vi "Main FPGA 5-axis with 5AxisLimitU8.vi"() -> ()   [LabVIEW 2013]
uses:
  <vilib>/Motion/MotorControl/_s/nism.interpretControlRegister.stateTransition.ctl
  <vilib>/Platform/TimedLoop/XDataNode/timing_clust.ctl
  <vilib>/Platform/TimedLoop/XDataNode/nitl_modes.ctl
  <vilib>/Platform/TimedLoop/XDataNode/wakeup.ctl
  <vilib>/Motion/MotorControl/_s/nism.digitalInputs.portA.ctl
  <vilib>/rvi/Emulation/niFpgaSctlEmulationGetInTimedLoop.vi
  <vilib>/rvi/Emulation/niFpgaEmulationReportErrorSimple.vi
  <vilib>/rvi/Emulation/niFpgaGetClockAttributes.vi
  <vilib>/rvi/Emulation/niFpgaCriticalErrorInLSC.vi
  Global FPGA.vi
  <vilib>/rvi/eio/common/nirviEmuTemplateMethod_errors.vi
  <vilib>/Motion/SoftMotion/Synchronization/nism.rioScan.generateSyncScan.vi
  <vilib>/rvi/Emulation/niFpgaProcessEmulError.vi
  <vilib>/Motion/MotorControl/_s/nism.interpretControlRegister.indexed.vi
  <vilib>/Motion/MotorControl/_s/nism.generateStatusRegister.indexed.vi
  <vilib>/Motion/MotorControl/_s/nism.mdo.read.positionLoopSyncData.vi
  <vilib>/Motion/MotorControl/_s/nism.mdo.read.splineData.vi
  <vilib>/Motion/MotorControl/_s/nism.splineInterpolation.fxp.3.index.vi
  <vilib>/Motion/MotorControl/_s/nism.mdo.handler.indexed.vi
  <vilib>/Motion/MotorControl/_s/nism.interpretDIOControl.portA.single.2.vi
  <vilib>/Motion/MotorControl/_s/nism.generateDIOStatus.portA.single.vi
  <vilib>/Platform/TimedLoop/XDataNode/XDataNode.xnode
  <vilib>/eio/EIONode/EIONode.xnode
  <vilib>/Motion/MotorControl/NI_SoftMotion_MotorControlIP.lvlib
  <vilib>/Platform/TimedLoop/XDataNode/XDNodeRunTimeDep.lvlib
  <vilib>/Motion/SoftMotion/Synchronization/NI_SoftMotion_Synchronization.lvlib
panel:
  in  "Axis Digital Input":u8[](array[numeric])=[0, 0, 0, 0, 0]
  out "Axis Positions":fxp<+/-,64,32>[](array[numeric])
  in  "STEP or CW? (T=STEP)":bool
  out "Drive Enable":bool[](array[boolean])
  in  "Enable Watchdog":bool
  in  "Pet Watchdog":bool
  in  "Watchdog Timeout Period (ticks)":u64=40000000 format="%.0p"
  out "Watchdog Timed Out?":bool
  out "Time Since Last Pet":u64
  in  "Enable value":bool
  in  "Drive Enable override?":bool
  out "State":T1=enum."Start --> Initializing" caption="state transition"
  in  "Sync Value":bool
  in  "Sync Enable override?":bool
  in  "Invert direction?":bool
  out "Sync is Fault":bool
  out "Sync is Locked":bool
  in  "minimum pulse":u16=40
  # "Synchronization Loop"
  # "Control Status Loop"
  # "Notes: \n1. This VI provides the communication interface between the NI SoftMotion Engine and the LabVIEW FPGA Module. You must compile this VI for a specific FPGA target before use. After compiling, run the VI before running any of the Express VI examples. For information on moving this example to another FPGA target, refer to ni.com/info and enter info code fpgaex.\n\n2. Only use the Reset Axis button if you are unable to communicate with the axis by any other means. This button resets the device state machine and other VIs to a known state. After resetting the axis, switch the NI Scan Engine from Active Mode to Configuration Mode, then back to Active Mode, before attempting to enable the axis."
  # "(These two buttons \nare for testing\npurposes.)"
  # "(These two buttons \nare for testing\npurposes.)"
  # "Step/Direction Loop"
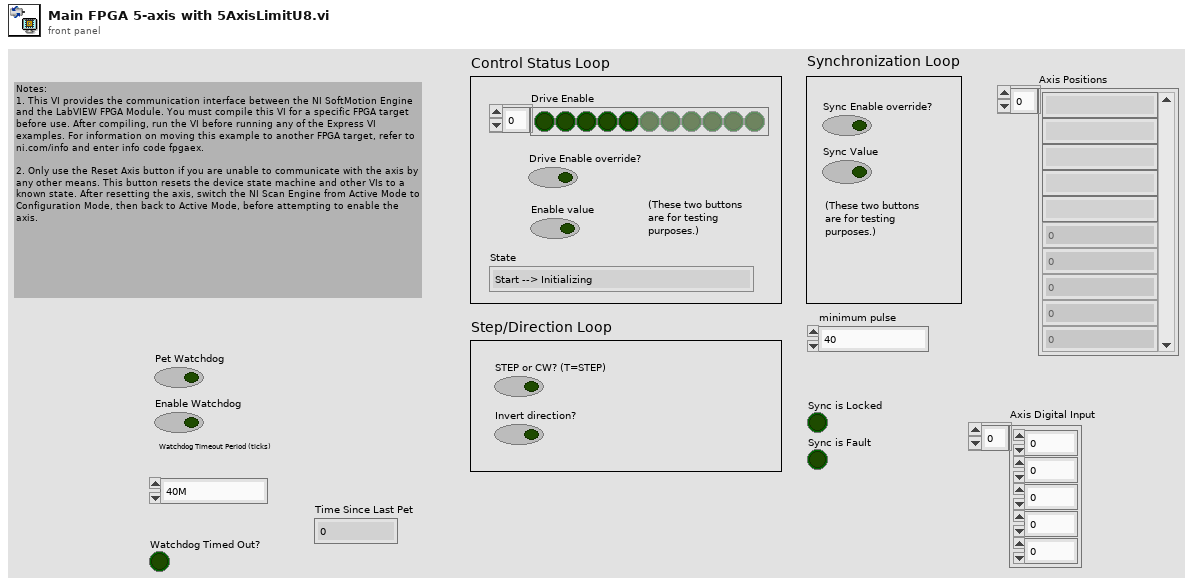
[diagram p1: front panel]
types:
  T1 = typedef "NI_SoftMotion_MotorControlIP.lvlib/nism.interpretControlRegister.stateTransition.ctl" = enum8{"Invalid", "Start --> Initializing", "Initializing --> Disabled", "Disabled --> Ready To Switch On", "Ready To Switch On --> Switched On", "Ready To Switch On --> Disable", "Switched On --> Operation Enable", "Switched On --> Ready To Switch On", "Switched On --> Disabled", "Operation Enable --> Switched On", "Operation Enable --> Ready To Switch On", "Operation Enable --> Disabled", "Fault --> Disabled", "Any --> Fault", "None"}
  T2 = typedef "NI_SoftMotion_MotorControlIP.lvlib/nism.mdo.splineData.ctl" = cluster{"spline type":T3, "traj per/spline per":u16, "spline per/traj per":fxp<+,32,0>}
  T3 = typedef "nism.splineInterpolation.type.ctl" = u16
  T4 = typedef "NI_SoftMotion_Synchronization.lvlib/nism.softmotionScan.timerConfig.ctl" = cluster{"Target Period (clocks)":u16, "Host Period / Target Period":u16}
  T5 = typedef "NI_SoftMotion_MotorControlIP.lvlib/nism.digitalInputs.portA.ctl" = cluster{"reverse limit":bool, "forward limit":bool, "home switch":bool, "digital input 0":bool, "digital input 1":bool, "digital input 2":bool, "digital input 3":bool}
  T6 = typedef "NI_SoftMotion_MotorControlIP.lvlib/nism.dio.portA.config.2.ctl" = cluster{"digital filter (us)":u16[], "safe state":enum16{"Low", "High", "No Change"}[]}
  T7 = typedef "NI_SoftMotion_Synchronization.lvlib/nism.softmotionScan.timerControl.ctl" = cluster{"SM Scan":bool, "SM Scan Count":u32, "SM Scan Enabled":bool}
  T8 = typedef "XDNodeRunTimeDep.lvlib/timing_clust.ctl" = cluster{"Expected End [f-1]":u64, "Actual End [f-1]":u64, "Finished Late? [f-1]":bool, "Expected End [i-1]":u64, "Actual End [i-1]":u64, "Finished Late? [i-1]":bool, "Expected Start [i]":u64, "Actual Start [i]":u64, "Expected Start [f]":u64, "Actual Start [f]":u64, "Source Name":string, "Structure Name":string, "Period":i64, "Deadline":i64, "Offset":i64, "Start":i64, "Priority":i32, "Timeout":i32, "Mode":T9, "Wakeup Reason":T10, "Error":errorcluster, "Source Type":string, "Secondary Source Type":string, "Global End Time":u64, "Global Start Time":u64, "Frame Duration":u64, "Iteration Duration":u64, "Assigned CPU":i32, "I/O Scan Engine Mode":u32}
  T9 = typedef "XDNodeRunTimeDep.lvlib/nitl_modes.ctl" = enum32{"No Change", "Process missed periods, maintain original phase", "Discard missed periods, maintain original phase", "Process missed periods, ignore original phase", "Discard missed periods, ignore original phase"}
  T10 = typedef "XDNodeRunTimeDep.lvlib/wakeup.ctl" = enum32{"Normal", "Aborted", "Asynchronous wakeup", "Timing source error", "Timed loop error", "Timeout"}
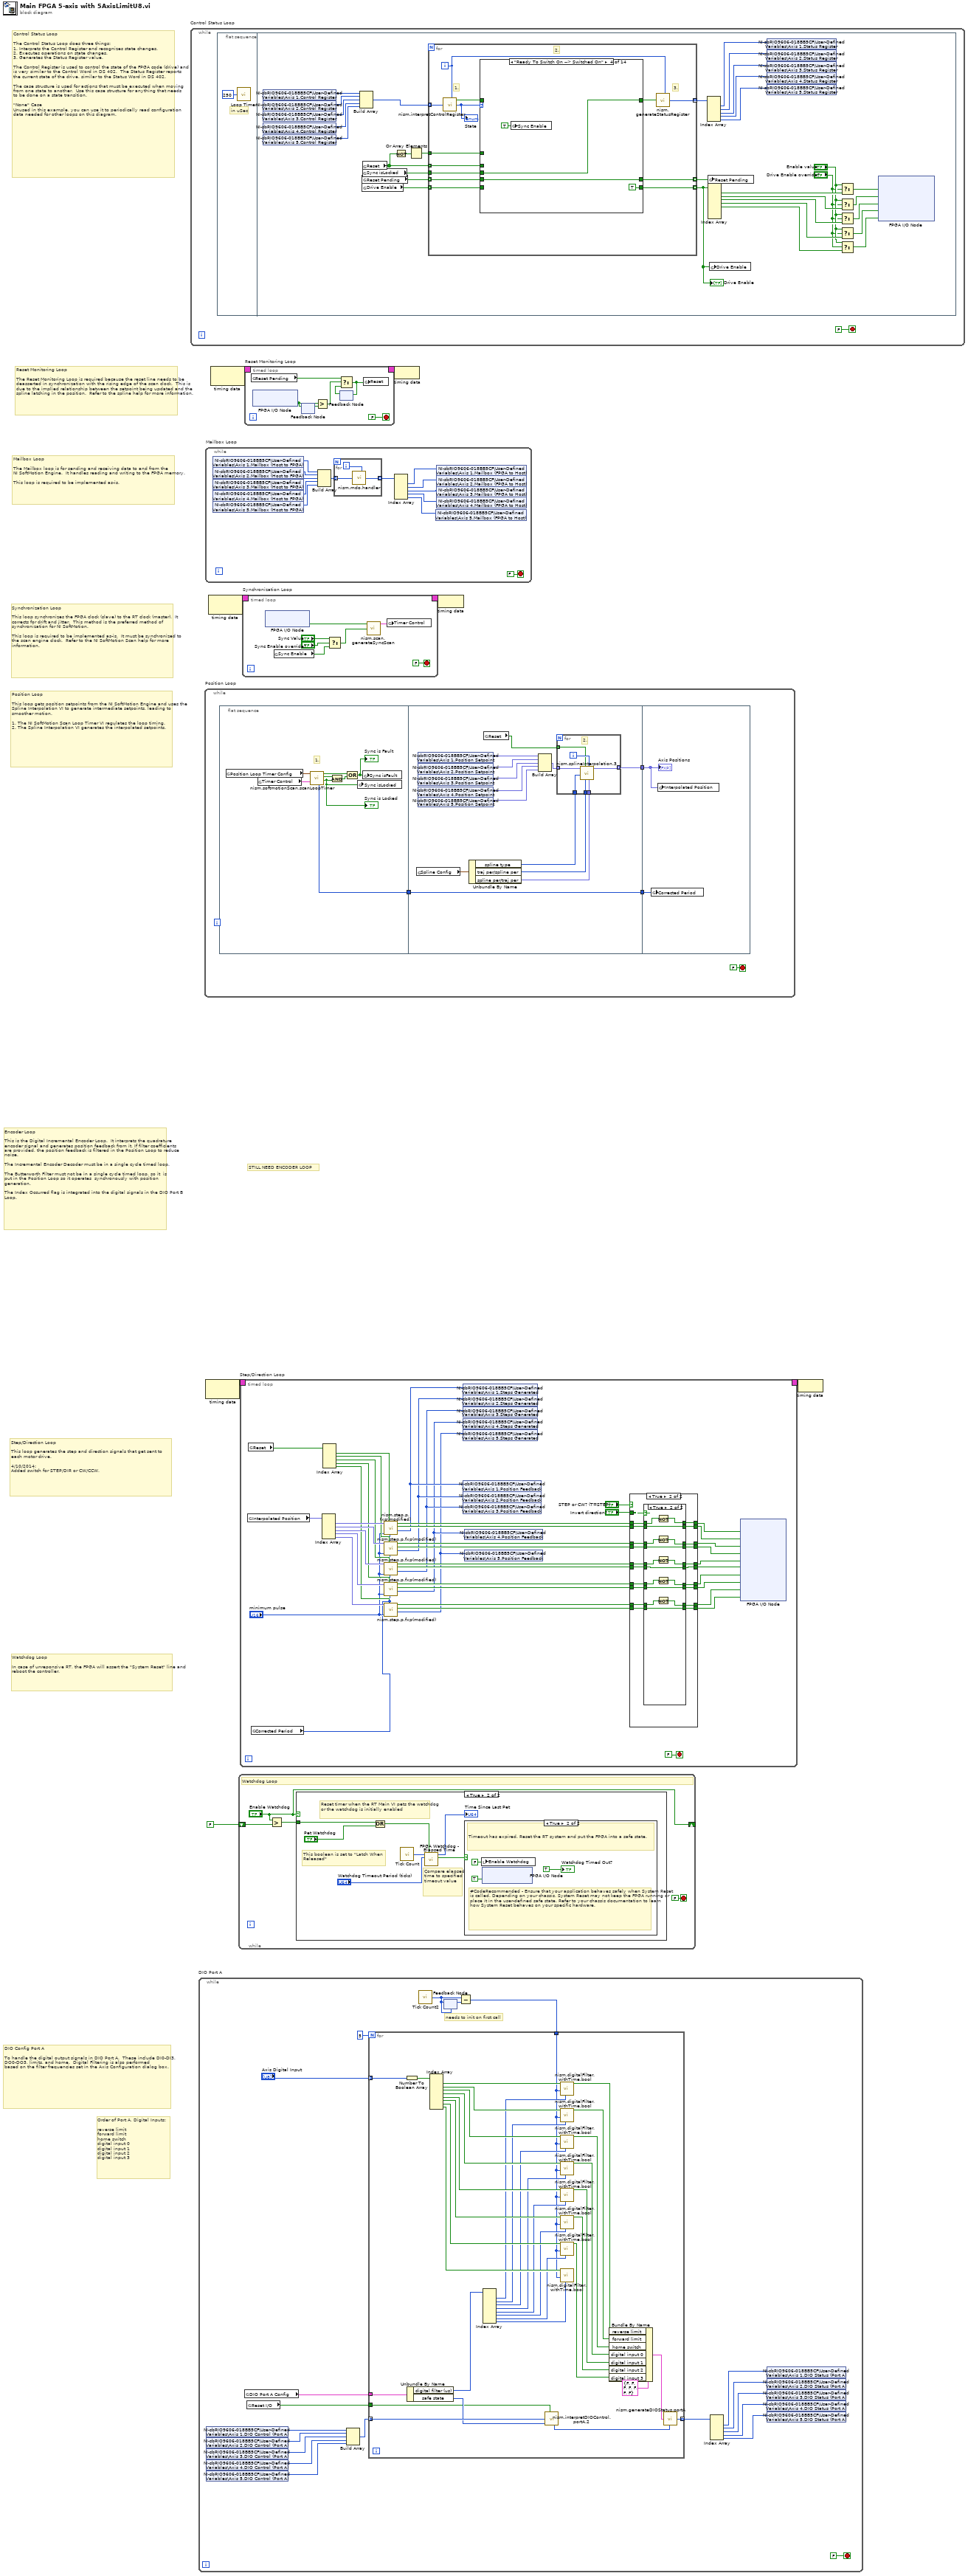
[diagram p0: block diagram]
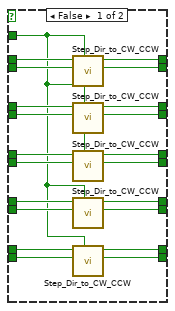
[diagram p4: hidden frame]
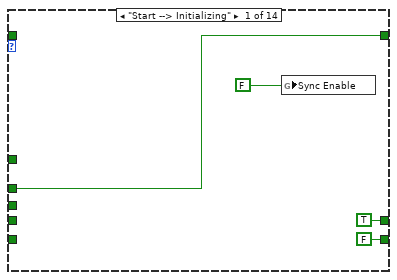
[diagram p6: hidden frame]
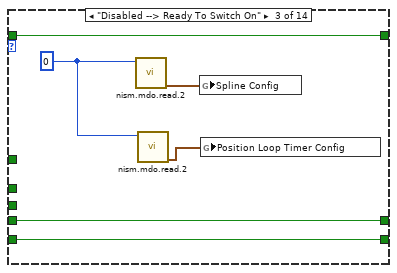
[diagram p8: hidden frame]
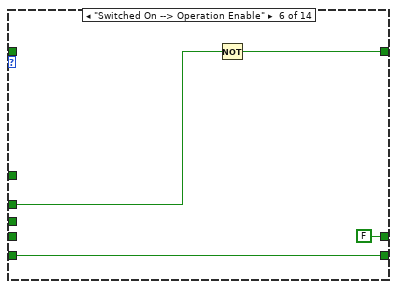
[diagram p10: hidden frame]
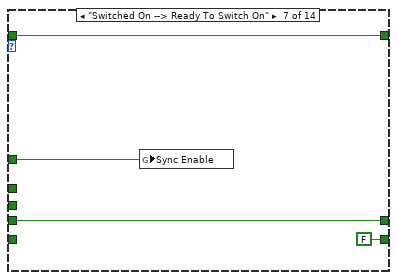
[diagram p11: hidden frame]
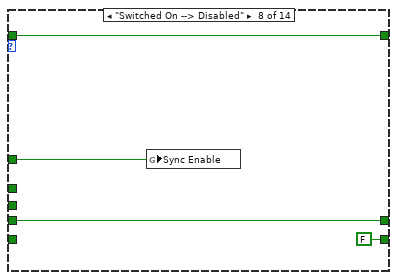
[diagram p12: hidden frame]
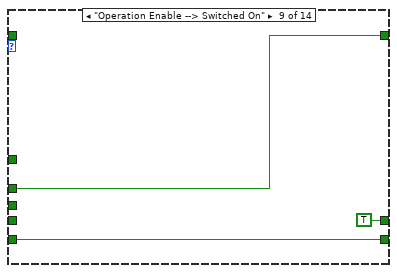
[diagram p13: hidden frame]
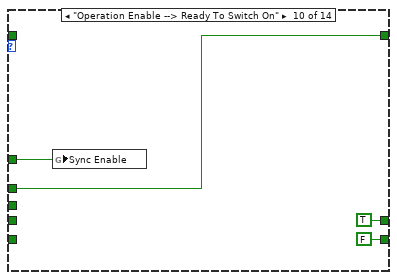
[diagram p14: hidden frame]
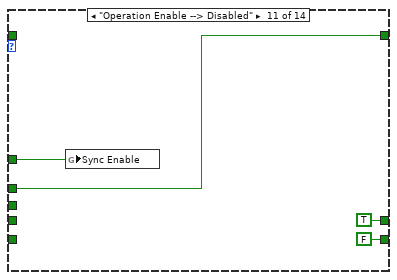
[diagram p15: hidden frame]
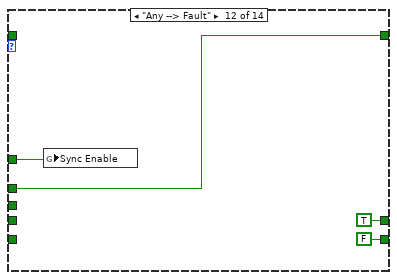
[diagram p16: hidden frame]
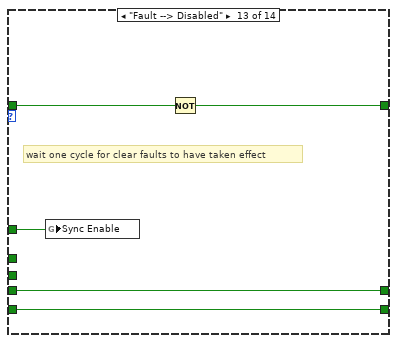
[diagram p17: hidden frame]
diagram:
  # "STILL NEED ENCODER LOOP"
  # "DIO Config Port A\n\nTo handle the digital output signals in DIO Port A.  These include DI0-DI3, DO0-DO3, limits, and home.  Digital Filtering is also performed\nbased on the filter frequencies set in the Axis Configuration dialog box."
  # "Order of Port A, Digital Inputs:\n\nreverse limit\nforward limit\nhome switch\ndigital input 0\ndigital input 1\ndigital input 2\ndigital input 3"
  # "Encoder Loop\n\nThis is the Digital Incremental Encoder Loop.  It interprets the quadrature encoder signal and generates position feedback from it. If filter coefficients are provided, the position feedback is filtered in the Position Loop to reduce noise.\n\nThe Incremental Encoder Decoder must be in a single cycle timed loop.\n\nThe Butterworth Filter must not be in a single cycle timed loop, so it  is\nput in the Position Loop so it operates  synchronously with position generation.\n\nThe Index Occurred flag is integrated into the digital signals in the DIO Port B Loop."
  # "Watchdog Loop\n\nIn case of unreponsive RT, the FPGA will assert the \"System Reset\" line and reboot the controller."
  # "Step/Direction Loop\n\nThis loop generates the step and direction signals that get sent to \neach motor drive.\n\n4/10/2014:\nAdded switch for STEP/DIR or CW/CCW."
  # "Position Loop\n\nThis loop gets position setpoints from the NI SoftMotion Engine and uses the Spline Interpolation VI to generate intermediate setpoints, leading to smoother motion.\n\n1. The NI SoftMotion Scan Loop Timer VI regulates the loop timing. \n2. The Spline Interpolation VI generates the interpolated setpoints."
  # "Synchronization Loop\n\nThis loop synchronizes the FPGA clock (slave) to the RT clock (master).  It corrects for drift and jitter.  This method is the preferred method of synchronization for NI SoftMotion.\n\nThis loop is required to be implemented as-is.  It must be synchronized to the scan engine clock.  Refer to the NI SoftMotion Scan help for more information."
  # "Mailbox Loop\n\nThe Mailbox loop is for sending and receiving data to and from the \nNI SoftMotion Engine.  It handles reading and writing to the FPGA memory.\n\nThis loop is required to be implemented as-is."
  # "Reset Monitoring Loop\n\nThe Reset Monitoring Loop is required because the reset line needs to be deasserted in synchronization with the rising edge of the scan clock.  This is due to the implied relationship between the setpoint being updated and the spline latching in the position.  Refer to the spline help for more information."
  # "Control Status Loop\n\nThe Control Status Loop does three things:\n1. Interprets the Control Register and recognizes state changes.\n2. Executes operations on state changes.\n3. Generates the Status Register value.\n\nThe Control Register is used to control the state of the FPGA code (drive) and is very similar to the Control Word in DS 402.  The Status Register reports the current state of the drive, similar to the Status Word in DS 402.\n\nThe case structure is used for actions that must be executed when moving from one state to another.  Use this case structure for anything that needs to be done on a state transition.\n\n\"None\" Case\nUnused in this example, you can use it to periodically read configuration data needed for other loops on this diagram."
  n1 = while "Control Status Loop" {
    stop <- FALSE stop-if-true
    n2 = flat-sequence {
      frame #0 {
        # "in uSec"
        n3 = call "Loop Timer"("Count(uSec)"=u32 250) -> ()  [unwired: 1 out]
      }
      frame #1 {
        n4 = shared-variable "NI-sbRIO9606-018BB5CF\\User-Defined Variables\\Axis 1.Control Register"() -> (w31:u32)  [unwired: 1 in, 1 out]
        n5 = shared-variable "NI-sbRIO9606-018BB5CF\\User-Defined Variables\\Axis 2.Control Register"() -> (w30:u32)  [unwired: 1 in, 1 out]
        n6 = shared-variable "NI-sbRIO9606-018BB5CF\\User-Defined Variables\\Axis 3.Control Register"() -> (w29:u32)  [unwired: 1 in, 1 out]
        n7 = shared-variable "NI-sbRIO9606-018BB5CF\\User-Defined Variables\\Axis 4.Control Register"() -> (w28:u32)  [unwired: 1 in, 1 out]
        n8 = shared-variable "NI-sbRIO9606-018BB5CF\\User-Defined Variables\\Axis 5.Control Register"() -> (w27:u32)  [unwired: 1 in, 1 out]
        n9 = Build Array(w31, w30, w29, w28, w27) -> (w40:u32[])
        n10 = global read "Global FPGA.vi" "Reset Pending"() -> (w35:bool[])
        n11 = global read "Global FPGA.vi" "Drive Enable"() -> (w34:bool[])
        n12 = global read "Global FPGA.vi" "Reset"() -> (w36:bool[])
        n13 = global read "Global FPGA.vi" "Sync isLocked"() -> (w41:bool)
        n14 = Not(x=w36) -> (.not. x?=w38:bool[])
        n15 = Or Array Elements(Boolean array=w38) -> (logical OR=w37:bool)
        n16 = for {
          tunnel: w36 -> [w49] mode=indexing
          tunnel: w41 -> [w48]
          tunnel: w40 -> [w50] mode=indexing
          tunnel: [w47] -> w32 mode=indexing
          tunnel: [w46] -> w39 mode=indexing
          tunnel: [w45] -> w33 mode=indexing
          tunnel: w37 -> [w44]
          tunnel: w35 -> [w43] mode=indexing
          tunnel: w34 -> [w42] mode=indexing
          i -> [w51]
          # "3."
          # "2."
          # "1."
          n17 = call-poly <vilib>:"nism.interpretControlRegister.vi"("control register"=w50, "axis index"=w51) -> ("transition occurred"=w52:bool, "state transition"=w53:T1)  [unwired: 6 in]
          "State" <- w53
          n18 = case shown="\"Ready To Switch On --> Switched On\"" w53 {
            tunnel: w52 -> [_ w61 w67 _ w74 _ w82 w86 _ _ _ _ w106 _]
            tunnel: [w58 w61 w67 w69 w74 w78 w82 w86 w88 w91 w95 w99 w105 _] -> w54
            tunnel: w49 -> [w58 _ _ _ _ w77 _ _ w88 w91 w95 w99 _ _]
            tunnel: w48 -> [_ _ _ w69 _ _ _ _ _ _ _ _ _ _]
            tunnel: [TRUE ("Write.Reset Pending") w60 w63 w68 w73 FALSE ("Write.Reset Pending") w79 w83 TRUE ("Write.Reset Pending") TRUE ("Write.Reset Pending") TRUE ("Write.Reset Pending") TRUE ("Write.Reset Pending") w103 w108] -> w46
            tunnel: [FALSE ("Write.Drive Enable") w59 w62 TRUE ("Write.Drive Enable") w72 w75 FALSE ("Write.Drive Enable") FALSE ("Write.Drive Enable") w87 FALSE ("Write.Drive Enable") FALSE ("Write.Drive Enable") FALSE ("Write.Drive Enable") w102 w107] -> w45
            tunnel: w44 -> [_ _ _ _ _ _ w80 w84 _ w90 w94 w98 w104 _]
            tunnel: w43 -> [_ w60 w63 w68 w73 _ w79 w83 _ _ _ _ w103 w108]
            tunnel: w42 -> [_ w59 w62 _ w72 w75 _ _ w87 _ _ _ w102 w107]
            frame "Start --> Initializing" {
              n19 = global write "Global FPGA.vi" "Sync Enable"(FALSE ("Sync Enable")) -> ()
            }
            frame "Initializing --> Disabled" {
            }
            frame "Disabled --> Ready To Switch On" {
              w65 = 0 ("axis index")
              n20 = call-poly <vilib>:"nism.mdo.read.2.vi"("axis index"=w65) -> ("spline"=w66:T2)  [unwired: 10 in]
              n21 = call-poly <vilib>:"nism.mdo.read.2.vi"("axis index"=w65) -> ("position loop sync"=w64:T4)  [unwired: 10 in]
              n22 = global write "Global FPGA.vi" "Spline Config"(w66) -> ()
              n23 = global write "Global FPGA.vi" "Position Loop Timer Config"(w64) -> ()
            }
            frame "Ready To Switch On --> Switched On" {
              n24 = global write "Global FPGA.vi" "Sync Enable"(TRUE ("Sync Enable")) -> ()
            }
            frame "Ready To Switch On --> Disable" {
            }
            frame "Switched On --> Operation Enable" {
              n25 = Not(x=w77) -> (.not. x?=w78:bool)
            }
            frame "Switched On --> Ready To Switch On" {
              n26 = global write "Global FPGA.vi" "Sync Enable"(w80) -> ()
            }
            frame "Switched On --> Disabled" {
              n27 = global write "Global FPGA.vi" "Sync Enable"(w84) -> ()
            }
            frame "Operation Enable --> Switched On" {
            }
            frame "Operation Enable --> Ready To Switch On" {
              n28 = global write "Global FPGA.vi" "Sync Enable"(w90) -> ()
            }
            frame "Operation Enable --> Disabled" {
              n29 = global write "Global FPGA.vi" "Sync Enable"(w94) -> ()
            }
            frame "Any --> Fault" {
              n30 = global write "Global FPGA.vi" "Sync Enable"(w98) -> ()
            }
            frame "Fault --> Disabled" {
              # "wait one cycle for clear faults to have taken effect"
              n31 = global write "Global FPGA.vi" "Sync Enable"(w104) -> ()
              n32 = Not(x=w106) -> (.not. x?=w105:bool)
            }
            frame "None", Default {
            }
          }
          n33 = call-poly <vilib>:"nism.generateStatusRegister.vi"("transition success"=w54, "axis index"=w51) -> ("status register"=w47:u32)  [unwired: 7 in]
        }
        "Drive Enable" <- w33
        n34 = Index Array(array=w32) -> (element #1=w26:u32, element #2=w25:u32, element #3=w24:u32, element #4=w23:u32, element #5=w22:u32)  [unwired: 5 in]
        n35 = global write "Global FPGA.vi" "Reset Pending"(w39) -> ()
        n36 = Index Array(array=w33) -> (element #1=w21:bool, element #2=w19:bool, element #3=w17:bool, element #4=w15:bool, element #5=w13:bool)  [unwired: 8 in, 3 out]
        n37 = global write "Global FPGA.vi" "Drive Enable"(w33) -> ()
        n38 = shared-variable "NI-sbRIO9606-018BB5CF\\User-Defined Variables\\Axis 1.Status Register"(w26) -> ()  [unwired: 1 in, 1 out]
        n39 = shared-variable "NI-sbRIO9606-018BB5CF\\User-Defined Variables\\Axis 2.Status Register"(w25) -> ()  [unwired: 1 in, 1 out]
        n40 = shared-variable "NI-sbRIO9606-018BB5CF\\User-Defined Variables\\Axis 3.Status Register"(w24) -> ()  [unwired: 1 in, 1 out]
        n41 = shared-variable "NI-sbRIO9606-018BB5CF\\User-Defined Variables\\Axis 4.Status Register"(w23) -> ()  [unwired: 1 in, 1 out]
        n42 = shared-variable "NI-sbRIO9606-018BB5CF\\User-Defined Variables\\Axis 5.Status Register"(w22) -> ()  [unwired: 1 in, 1 out]
        n43 = Select(t="Enable value", s="Drive Enable override?", f=w21) -> (s? t:f=w20:bool)
        n44 = Select(t="Enable value", s="Drive Enable override?", f=w19) -> (s? t:f=w18:bool)
        n45 = Select(t="Enable value", s="Drive Enable override?", f=w17) -> (s? t:f=w16:bool)
        n46 = Select(t="Enable value", s="Drive Enable override?", f=w15) -> (s? t:f=w14:bool)
        n47 = Select(t="Enable value", s="Drive Enable override?", f=w13) -> (s? t:f=w12:bool)
        n48 = xnode "FPGA I/O Node"("Axis1_Servo On"=w20, "Axis2_Servo On"=w18, "Axis3_Servo On"=w16, "Axis4_Servo On"=w14, "Axis5_Servo On"=w12) -> ()  [unwired: 5 in, 5 out]
      }
    }
  }
  n49 = while "DIO Port A" {
    stop <- FALSE stop-if-true
    # "needs to init on first call"
    n50 = shared-variable "NI-sbRIO9606-018BB5CF\\User-Defined Variables\\Axis 1.DIO Control (Port A)"() -> (w123:u32)  [unwired: 1 in, 1 out]
    n51 = shared-variable "NI-sbRIO9606-018BB5CF\\User-Defined Variables\\Axis 2.DIO Control (Port A)"() -> (w122:u32)  [unwired: 1 in, 1 out]
    n52 = shared-variable "NI-sbRIO9606-018BB5CF\\User-Defined Variables\\Axis 3.DIO Control (Port A)"() -> (w121:u32)  [unwired: 1 in, 1 out]
    n53 = shared-variable "NI-sbRIO9606-018BB5CF\\User-Defined Variables\\Axis 4.DIO Control (Port A)"() -> (w120:u32)  [unwired: 1 in, 1 out]
    n54 = shared-variable "NI-sbRIO9606-018BB5CF\\User-Defined Variables\\Axis 5.DIO Control (Port A)"() -> (w119:u32)  [unwired: 1 in, 1 out]
    n55 = global read "Global FPGA.vi" "DIO Port A Config"() -> (w127:T6)
    n56 = global read "Global FPGA.vi" "Reset I/O"() -> (w126:bool)
    n57 = Build Array(w123, w122, w121, w120, w119) -> (w118:u32[])
    n58 = call "Tick Count2"() -> ("Tick Count(uSec)"=w111:u16)
    n59 = feedback #1(w111) -> (w110:u16)
    n60 = feedback-in #1(w111) -> ()
    n61 = Subtract(x=w111, y=w110) -> (x-y=w109:u16)
    n62 = for {
      N: 5 -> [_]
      tunnel: [w162] -> w112 mode=indexing
      tunnel: w118 -> [w161] mode=indexing
      tunnel: w127 -> [w158]
      tunnel: w126 -> [w156]
      tunnel: "Axis Digital Input" -> [w130] mode=indexing
      tunnel: w109 -> [w129]
      n63 = Number To Boolean Array(number=w130) -> (Boolean array=w155:bool[])
      n64 = Unbundle By Name(w158) -> ("digital filter (us)"=w138:u16[], "safe state"=w157:enum16{"Low", "High", "No Change"}[])
      n65 = Index Array(array=w155) -> (element #1=w154:bool, element #2=w147:bool, element #3=w148:bool, element #4=w149:bool, element #5=w150:bool, element #6=w151:bool, element #7=w152:bool, element #8=w153:bool)  [unwired: 8 in]
      n66 = Index Array(array=w138) -> (element #1=w139:u16, element #2=w140:u16, element #3=w141:u16, element #4=w142:u16, element #5=w143:u16, element #6=w144:u16, element #7=w145:u16, element #8=w146:u16)  [unwired: 8 in]
      n67 = call-poly <vilib>:"nism.interpretDIOControl.portA.2.vi"("reset"=w156, "dio control(port a)"=w161, "safe state"=w157) -> ("reset latches"=w163:u8)  [unwired: 5 in, 1 out]
      n68 = call <vilib>:"nism.digitalFilter.withTime.bool.vi"("filter value"=w139, "delta time"=w129, "input signal"=w154) -> ("output signal"=w137:bool)  [unwired: 8 in]
      n69 = call <vilib>:"nism.digitalFilter.withTime.bool.vi"("filter value"=w140, "delta time"=w129, "input signal"=w147) -> ("output signal"=w136:bool)  [unwired: 8 in]
      n70 = call <vilib>:"nism.digitalFilter.withTime.bool.vi"("filter value"=w141, "delta time"=w129, "input signal"=w148) -> ("output signal"=w135:bool)  [unwired: 8 in]
      n71 = call <vilib>:"nism.digitalFilter.withTime.bool.vi"("filter value"=w142, "delta time"=w129, "input signal"=w149) -> ("output signal"=w134:bool)  [unwired: 8 in]
      n72 = call <vilib>:"nism.digitalFilter.withTime.bool.vi"("filter value"=w143, "delta time"=w129, "input signal"=w150) -> ("output signal"=w133:bool)  [unwired: 8 in]
      n73 = call <vilib>:"nism.digitalFilter.withTime.bool.vi"("filter value"=w144, "delta time"=w129, "input signal"=w151) -> ("output signal"=w132:bool)  [unwired: 8 in]
      n74 = call <vilib>:"nism.digitalFilter.withTime.bool.vi"("filter value"=w145, "delta time"=w129, "input signal"=w152) -> ("output signal"=w131:bool)  [unwired: 8 in]
      n75 = call <vilib>:"nism.digitalFilter.withTime.bool.vi"("filter value"=w146, "delta time"=w129, "input signal"=w153) -> ()  [unwired: 8 in, 1 out]
      n76 = Bundle By Name(cluster=T5 {"reverse limit"=FALSE, "forward limit"=FALSE, "home switch"=FALSE, "digital input 0"=FALSE, "digital input 1"=FALSE, "digital input 2"=FALSE, "digital input 3"=FALSE} ("$(driveInterface.digitalInputs.shortName)"), "reverse limit"=w137, "forward limit"=w136, "home switch"=w135, "digital input 0"=w134, "digital input 1"=w133, "digital input 2"=w132, "digital input 3"=w131) -> (w159:T5)
      n77 = call-poly <vilib>:"nism.generateDIOStatus.portA.vi"("digital inputs"=w159, "reset latches"=w163) -> ("dio status(port a)"=w162:u32)  [unwired: 7 in]
    }
    n78 = Index Array(array=w112) -> (element #1=w117:u32, element #2=w116:u32, element #3=w115:u32, element #4=w114:u32, element #5=w113:u32)  [unwired: 5 in]
    n79 = shared-variable "NI-sbRIO9606-018BB5CF\\User-Defined Variables\\Axis 1.DIO Status (Port A)"(w117) -> ()  [unwired: 1 in, 1 out]
    n80 = shared-variable "NI-sbRIO9606-018BB5CF\\User-Defined Variables\\Axis 2.DIO Status (Port A)"(w116) -> ()  [unwired: 1 in, 1 out]
    n81 = shared-variable "NI-sbRIO9606-018BB5CF\\User-Defined Variables\\Axis 3.DIO Status (Port A)"(w115) -> ()  [unwired: 1 in, 1 out]
    n82 = shared-variable "NI-sbRIO9606-018BB5CF\\User-Defined Variables\\Axis 4.DIO Status (Port A)"(w114) -> ()  [unwired: 1 in, 1 out]
    n83 = shared-variable "NI-sbRIO9606-018BB5CF\\User-Defined Variables\\Axis 5.DIO Status (Port A)"(w113) -> ()  [unwired: 1 in, 1 out]
  }
  n84 = while "Position Loop" {
    stop <- FALSE stop-if-true
    n85 = flat-sequence {
      tunnel: [w168] -> w164
      tunnel: [w182] -> w166
      tunnel: [w181] -> w165
      tunnel: w164 -> [w181]
      tunnel: w166 -> [w196]
      tunnel: w165 -> [w197]
      frame #0 {
        # "1."
        n86 = global read "Global FPGA.vi" "Position Loop Timer Config"() -> (w170:T4)
        n87 = global read "Global FPGA.vi" "Timer Control"() -> (w169:T7)
        n88 = call <vilib>:"nism.softmotionScan.scanLoopTimer.vi"("Timer Control"=w169, "Timer Config"=w170) -> ("Scan Running?"=w172:bool, "Finished Late?"=w174:bool, "Fault Occurred?"=w175:bool, "Corrected Period"=w168:u16)  [unwired: 5 in, 1 out]
        "Sync is Locked" <- w172
        n89 = Compound Arithmetic op=AND(w174, w172) -> (w173:bool)
        n90 = Compound Arithmetic op=OR(w175, w173) -> (w171:bool)
        "Sync is Fault" <- w171
        n91 = global write "Global FPGA.vi" "Sync isLocked"(w172) -> ()
        n92 = global write "Global FPGA.vi" "Sync isFault"(w171) -> ()
      }
      frame #1 {
        n93 = global read "Global FPGA.vi" "Spline Config"() -> (w184:T2)
        n94 = shared-variable "NI-sbRIO9606-018BB5CF\\User-Defined Variables\\Axis 1.Position Setpoint"() -> (w180:fxp<+/-,64,32>)  [unwired: 1 in, 1 out]
        n95 = shared-variable "NI-sbRIO9606-018BB5CF\\User-Defined Variables\\Axis 2.Position Setpoint"() -> (w179:fxp<+/-,64,32>)  [unwired: 1 in, 1 out]
        n96 = shared-variable "NI-sbRIO9606-018BB5CF\\User-Defined Variables\\Axis 3.Position Setpoint"() -> (w178:fxp<+/-,64,32>)  [unwired: 1 in, 1 out]
        n97 = shared-variable "NI-sbRIO9606-018BB5CF\\User-Defined Variables\\Axis 4.Position Setpoint"() -> (w177:fxp<+/-,64,32>)  [unwired: 1 in, 1 out]
        n98 = shared-variable "NI-sbRIO9606-018BB5CF\\User-Defined Variables\\Axis 5.Position Setpoint"() -> (w176:fxp<+/-,64,32>)  [unwired: 1 in, 1 out]
        n99 = Unbundle By Name(w184) -> ("spline type"=w188:T3, "traj per/spline per"=w187:u16, "spline per/traj per"=w186:fxp<+,32,0>)
        n100 = global read "Global FPGA.vi" "Reset"() -> (w183:bool[])
        n101 = Build Array(w180, w179, w178, w177, w176) -> (w185:fxp<+/-,64,32>[])
        n102 = for {
          tunnel: w188 -> [w195]
          tunnel: w187 -> [w194]
          tunnel: w186 -> [w193]
          tunnel: w183 -> [w190] mode=indexing
          tunnel: w185 -> [w192] mode=indexing
          tunnel: [w189] -> w182 mode=indexing
          i -> [w191]
          # "2."
          n103 = call-poly <vilib>:"nism.splineInterpolation.3.vi"("1 / calls per sample"=w193, "index"=w191, "calls per sample"=w194, "reset"=w190, "spline type"=w195, "x"=w192) -> ("xi"=w189:fxp<+/-,64,32>)  [unwired: 5 in]
        }
      }
      frame #2 {
        n104 = global write "Global FPGA.vi" "Corrected Period"(w197) -> ()
        n105 = global write "Global FPGA.vi" "Interpolated Position"(w196) -> ()
        "Axis Positions" <- w196
      }
    }
  }
  n106 = while "Mailbox Loop" {
    stop <- FALSE stop-if-true
    n107 = shared-variable "NI-sbRIO9606-018BB5CF\\User-Defined Variables\\Axis 1.Mailbox (Host to FPGA)"() -> (w207:u64)  [unwired: 1 in, 1 out]
    n108 = shared-variable "NI-sbRIO9606-018BB5CF\\User-Defined Variables\\Axis 2.Mailbox (Host to FPGA)"() -> (w206:u64)  [unwired: 1 in, 1 out]
    n109 = shared-variable "NI-sbRIO9606-018BB5CF\\User-Defined Variables\\Axis 3.Mailbox (Host to FPGA)"() -> (w205:u64)  [unwired: 1 in, 1 out]
    n110 = shared-variable "NI-sbRIO9606-018BB5CF\\User-Defined Variables\\Axis 4.Mailbox (Host to FPGA)"() -> (w204:u64)  [unwired: 1 in, 1 out]
    n111 = shared-variable "NI-sbRIO9606-018BB5CF\\User-Defined Variables\\Axis 5.Mailbox (Host to FPGA)"() -> (w203:u64)  [unwired: 1 in, 1 out]
    n112 = Build Array(w207, w206, w205, w204, w203) -> (w209:u64[])
    n113 = for {
      tunnel: w209 -> [w213] mode=indexing
      tunnel: [w212] -> w208 mode=indexing
      i -> [w211]
      n114 = call-poly <vilib>:"nism.mdo.handler.vi"("mbox (host to fpga)"=w213, "axis index"=w211) -> ("mbox (fpga to host)"=w212:u64)  [unwired: 7 in]
    }
    n115 = Index Array(array=w208) -> (element #1=w202:u64, element #2=w201:u64, element #3=w200:u64, element #4=w199:u64, element #5=w198:u64)  [unwired: 5 in]
    n116 = shared-variable "NI-sbRIO9606-018BB5CF\\User-Defined Variables\\Axis 5.Mailbox (FPGA to Host)"(w198) -> ()  [unwired: 1 in, 1 out]
    n117 = shared-variable "NI-sbRIO9606-018BB5CF\\User-Defined Variables\\Axis 1.Mailbox (FPGA to Host)"(w202) -> ()  [unwired: 1 in, 1 out]
    n118 = shared-variable "NI-sbRIO9606-018BB5CF\\User-Defined Variables\\Axis 2.Mailbox (FPGA to Host)"(w201) -> ()  [unwired: 1 in, 1 out]
    n119 = shared-variable "NI-sbRIO9606-018BB5CF\\User-Defined Variables\\Axis 3.Mailbox (FPGA to Host)"(w200) -> ()  [unwired: 1 in, 1 out]
    n120 = shared-variable "NI-sbRIO9606-018BB5CF\\User-Defined Variables\\Axis 4.Mailbox (FPGA to Host)"(w199) -> ()  [unwired: 1 in, 1 out]
  }
  n121 = node-c288() -> (w7:T8)  [unwired: 1 in]
  n122 = node-c288() -> (w5:T8)  [unwired: 1 in]
  n123 = node-c288() -> (w3:T8)  [unwired: 1 in]
  n124 = while "RT Watchdog Loop" {
    shift-right: ["Enable Watchdog"] -> _
    shift-left: FALSE ("Enable RT Watchdog") -> [w217]
    stop <- FALSE stop-if-true
    # "Watchdog Loop"
    n125 = Greater?(x="Enable Watchdog", y=w217) -> (0:w214:bool)
    n126 = case shown="True" "Enable Watchdog" {
      tunnel: w214 -> [_ w220]
      frame False {
        # "This loop has to be explicitly enabled from the RT Main VI.  This reduces the possiblity of an endless reboot cycle."
      }
      frame True {
        # "This boolean is set to \"Latch When Released\""
        # "Compare elapsed time to specified timeout value"
        # "Reset timer when the RT Main VI pets the watchdog or the watchdog is initially enabled"
        n127 = Or(x=w220, y="Pet Watchdog") -> (x .or. y?=w219:bool)
        n128 = call "Tick Count"() -> ("Tick Count(Ticks)"=w223:u32)
        n129 = call "FPGA Watchdog - Elapsed Time.vi"("Reset"=w219, "Timeout Period"="Watchdog Timeout Period (ticks)", "Current Time"=w223) -> ("Timeout"=w218:bool, "Elapsed Time"=→"Time Since Last Pet":u64)  [unwired: 7 in]
        n130 = case shown="True" w218 {
          frame False {
            # "Timeout has not expired."
          }
          frame True {
            # "#CodeRecommended - Ensure that your application behaves safely when System Reset is called. Depending on your chassis, System Reset may not keep the FPGA running or place it in the user-defined safe state. Refer to your chassis documentation to learn how System Reset behaves on your specific hardware."
            # "Timeout has expired. Reset the RT system and put the FPGA into a safe state."
            n131 = local write "Enable Watchdog"(FALSE ("Enable RT Watchdog")) -> ()
            n132 = xnode "FPGA I/O Node"("System Reset"=TRUE ("RT Reset on Watchdog Failure?")) -> ()  [unwired: 1 in, 1 out]
            "Watchdog Timed Out?" <- TRUE ("Watchdog Timed Out?")
          }
        }
      }
    }
  }
  n133 = timed-loop "Step/Direction Loop" {
    timing: w7 -> [_]
    timing-out: [_] -> w6
    stop <- FALSE stop-if-true
    n134 = global read "Global FPGA.vi" "Interpolated Position"() -> (w268:fxp<+/-,64,32>[])
    n135 = global read "Global FPGA.vi" "Reset"() -> (w262:bool[])
    n136 = global read "Global FPGA.vi" "Corrected Period"() -> (w228:u16)
    n137 = Index Array(array=w268) -> (element #1=w267:fxp<+/-,64,32>, element #2=w266:fxp<+/-,64,32>, element #3=w265:fxp<+/-,64,32>, element #4=w264:fxp<+/-,64,32>, element #5=w263:fxp<+/-,64,32>)  [unwired: 5 in]
    n138 = Index Array(array=w262) -> (element #1=w261:bool, element #2=w260:bool, element #3=w259:bool, element #4=w258:bool, element #5=w257:bool)  [unwired: 5 in]
    n139 = call "nism.step.p.fxp(modified).vi"("calls per sample"=w228, "reset"=w261, "minimum pulse"="minimum pulse", "position setpoint"=w267) -> ("steps generated"=w233:i32, "step"=w255:bool, "direction"=w256:bool)  [unwired: 4 in, 1 out]
    n140 = call "nism.step.p.fxp(modified).vi"("calls per sample"=w228, "reset"=w260, "minimum pulse"="minimum pulse", "position setpoint"=w266) -> ("steps generated"=w232:i32, "step"=w253:bool, "direction"=w254:bool)  [unwired: 4 in, 1 out]
    n141 = call "nism.step.p.fxp(modified).vi"("calls per sample"=w228, "reset"=w259, "minimum pulse"="minimum pulse", "position setpoint"=w265) -> ("steps generated"=w231:i32, "step"=w251:bool, "direction"=w252:bool)  [unwired: 4 in, 1 out]
    n142 = call "nism.step.p.fxp(modified).vi"("calls per sample"=w228, "reset"=w258, "minimum pulse"="minimum pulse", "position setpoint"=w264) -> ("steps generated"=w230:i32, "step"=w249:bool, "direction"=w250:bool)  [unwired: 4 in, 1 out]
    n143 = call "nism.step.p.fxp(modified).vi"("calls per sample"=w228, "reset"=w257, "minimum pulse"="minimum pulse", "position setpoint"=w263) -> ("steps generated"=w229:i32, "step"=w247:bool, "direction"=w248:bool)  [unwired: 4 in, 1 out]
    n144 = shared-variable "NI-sbRIO9606-018BB5CF\\User-Defined Variables\\Axis 1.Steps Generated"(w233) -> ()  [unwired: 1 in, 1 out]
    n145 = shared-variable "NI-sbRIO9606-018BB5CF\\User-Defined Variables\\Axis 2.Steps Generated"(w232) -> ()  [unwired: 1 in, 1 out]
    n146 = shared-variable "NI-sbRIO9606-018BB5CF\\User-Defined Variables\\Axis 3.Steps Generated"(w231) -> ()  [unwired: 1 in, 1 out]
    n147 = shared-variable "NI-sbRIO9606-018BB5CF\\User-Defined Variables\\Axis 4.Steps Generated"(w230) -> ()  [unwired: 1 in, 1 out]
    n148 = shared-variable "NI-sbRIO9606-018BB5CF\\User-Defined Variables\\Axis 5.Steps Generated"(w229) -> ()  [unwired: 1 in, 1 out]
    n149 = shared-variable "NI-sbRIO9606-018BB5CF\\User-Defined Variables\\Axis 1.Position Feedback"(w233) -> ()  [unwired: 1 in, 1 out]
    n150 = shared-variable "NI-sbRIO9606-018BB5CF\\User-Defined Variables\\Axis 2.Position Feedback"(w232) -> ()  [unwired: 1 in, 1 out]
    n151 = shared-variable "NI-sbRIO9606-018BB5CF\\User-Defined Variables\\Axis 3.Position Feedback"(w231) -> ()  [unwired: 1 in, 1 out]
    n152 = shared-variable "NI-sbRIO9606-018BB5CF\\User-Defined Variables\\Axis 4.Position Feedback"(w230) -> ()  [unwired: 1 in, 1 out]
    n153 = shared-variable "NI-sbRIO9606-018BB5CF\\User-Defined Variables\\Axis 5.Position Feedback"(w229) -> ()  [unwired: 1 in, 1 out]
    n154 = case shown="True" "STEP or CW? (T=STEP)" {
      tunnel: w256 -> [w290 w310]
      tunnel: w255 -> [w289 w300]
      tunnel: w254 -> [w288 w308]
      tunnel: w253 -> [w287 w298]
      tunnel: w252 -> [w286 w306]
      tunnel: w251 -> [w285 w296]
      tunnel: w250 -> [w284 w304]
      tunnel: w249 -> [w283 w294]
      tunnel: w248 -> [w282 w302]
      tunnel: w247 -> [w281 w292]
      tunnel: "Invert direction?" -> [w270 w311]
      tunnel: [w280 w309] -> w245
      tunnel: [w279 w299] -> w236
      tunnel: [w278 w307] -> w244
      tunnel: [w277 w297] -> w243
      tunnel: [w276 w305] -> w242
      tunnel: [w275 w295] -> w241
      tunnel: [w274 w303] -> w240
      tunnel: [w273 w293] -> w239
      tunnel: [w272 w301] -> w238
      tunnel: [w271 w291] -> w237
      frame False {
        n155 = call "Step_Dir_to_CW_CCW.vi"("invert"=w270, "step"=w289, "direction"=w290) -> ("CCW"=w279:bool, "CW"=w280:bool)  [unwired: 7 in]
        n156 = call "Step_Dir_to_CW_CCW.vi"("invert"=w270, "step"=w287, "direction"=w288) -> ("CCW"=w277:bool, "CW"=w278:bool)  [unwired: 7 in]
        n157 = call "Step_Dir_to_CW_CCW.vi"("invert"=w270, "step"=w285, "direction"=w286) -> ("CCW"=w275:bool, "CW"=w276:bool)  [unwired: 7 in]
        n158 = call "Step_Dir_to_CW_CCW.vi"("invert"=w270, "step"=w283, "direction"=w284) -> ("CCW"=w273:bool, "CW"=w274:bool)  [unwired: 7 in]
        n159 = call "Step_Dir_to_CW_CCW.vi"("invert"=w270, "step"=w281, "direction"=w282) -> ("CCW"=w271:bool, "CW"=w272:bool)  [unwired: 7 in]
      }
      frame True {
        n160 = case shown="True" w311 {
          tunnel: w310 -> [w321 w336]
          tunnel: [w321 w335] -> w309
          tunnel: w308 -> [w319 w334]
          tunnel: [w319 w333] -> w307
          tunnel: w306 -> [w317 w332]
          tunnel: [w317 w331] -> w305
          tunnel: w304 -> [w315 w330]
          tunnel: [w315 w329] -> w303
          tunnel: w302 -> [w313 w328]
          tunnel: [w313 w327] -> w301
          tunnel: w300 -> [w320 w326]
          tunnel: [w320 w326] -> w299
          tunnel: w298 -> [w318 w325]
          tunnel: [w318 w325] -> w297
          tunnel: w296 -> [w316 w324]
          tunnel: [w316 w324] -> w295
          tunnel: w294 -> [w314 w323]
          tunnel: [w314 w323] -> w293
          tunnel: w292 -> [w312 w322]
          tunnel: [w312 w322] -> w291
          frame False {
          }
          frame True {
            n161 = Not(x=w336) -> (.not. x?=w335:bool)
            n162 = Not(x=w334) -> (.not. x?=w333:bool)
            n163 = Not(x=w332) -> (.not. x?=w331:bool)
            n164 = Not(x=w330) -> (.not. x?=w329:bool)
            n165 = Not(x=w328) -> (.not. x?=w327:bool)
          }
        }
      }
    }
    n166 = xnode "FPGA I/O Node"("Axis1_CW"=w245, "Axis1_CCW"=w236, "Axis2_CW"=w244, "Axis2_CCW"=w243, "Axis3_CW"=w242, "Axis3_CCW"=w241, "Axis4_CW"=w240, "Axis4_CCW"=w239, "Axis5_CW"=w238, "Axis5_CCW"=w237) -> ()  [unwired: 10 in, 10 out]
  }
  n167 = timed-loop "Synchronization Loop" {
    timing: w5 -> [_]
    timing-out: [_] -> w4
    stop <- FALSE stop-if-true
    n168 = xnode "FPGA I/O Node"() -> ("Scan Clock"=w343:bool)  [unwired: 1 in, 1 out]
    n169 = global read "Global FPGA.vi" "Sync Enable"() -> (w342:bool)
    n170 = Select(t="Sync Value", s="Sync Enable override?", f=w342) -> (s? t:f=w339:bool)
    n171 = call-poly <vilib>:"nism.scan.generateSyncScan.vi"("Scan Enable?"=w339, "Scan Clock"=w343) -> ("Timer Control"=w344:T7)  [unwired: 3 in]
    n172 = global write "Global FPGA.vi" "Timer Control"(w344) -> ()
  }
  n173 = timed-loop "Reset Monitoring Loop" {
    timing: w3 -> [_]
    timing-out: [_] -> w2
    stop <- FALSE stop-if-true
    n174 = global read "Global FPGA.vi" "Reset Pending"() -> (w350:bool[])
    n175 = xnode "FPGA I/O Node"() -> ("Scan Clock"=w349:bool)  [unwired: 1 in, 1 out]
    n176 = feedback-in #2(w349) -> ()
    n177 = feedback #2() -> (w348:bool)  [unwired: 1 in]
    n178 = Greater?(x=w349, y=w348) -> (0:w354:bool)
    n179 = feedback #3() -> (w353:bool[])  [unwired: 1 in]
    n180 = Select(t=w350, s=w354, f=w353) -> (s? t:f=w351:bool[])
    n181 = feedback-in #3(w351) -> ()
    n182 = global write "Global FPGA.vi" "Reset"(w351) -> ()
  }
  n183 = node-c288(w2) -> ()
  n184 = node-c288(w4) -> ()
  n185 = node-c288(w6) -> ()
